vi "Main.vi"() -> ()   [LabVIEW 2020]
doc: "Copyright (c) 2019, Labvolution Limited - www.labvolution.com\n\nThis software is distributed under the BSD 3-Clause License. For the full license please the LICENSE file or visit www.labvolution.com/license"
uses:
  callback-system-exec/CallbackSystemExec.vi
  callback-system-exec/callback-system-exec.lvlib
panel:
  in  "Abort command":bool
  out "Exit":bool
  in  "Execute command":bool
  in  "Working directory":path
  in  "Command":string(combo)
  out "Standard Error":string
  out "Standard Out":string
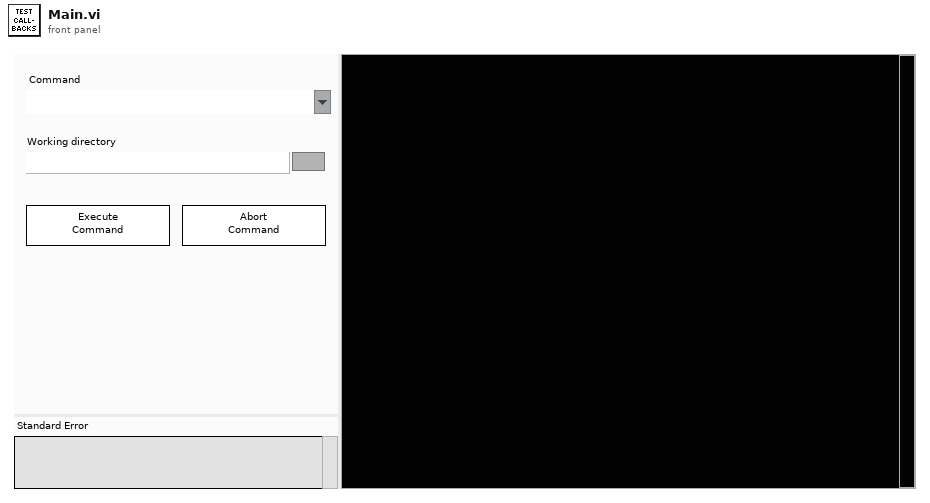
[diagram p1: front panel]
types:
  T1 = cluster{"Standard Out UE":refnum<user-event>, "Standard Error UE":refnum<user-event>, "Exited UE":refnum<user-event>}
  T2 = enum32{"invalid app kind", "Development System", "Run Time System", "Student Edition", "Embedded LabVIEW", "Evaluation", "Custom"}
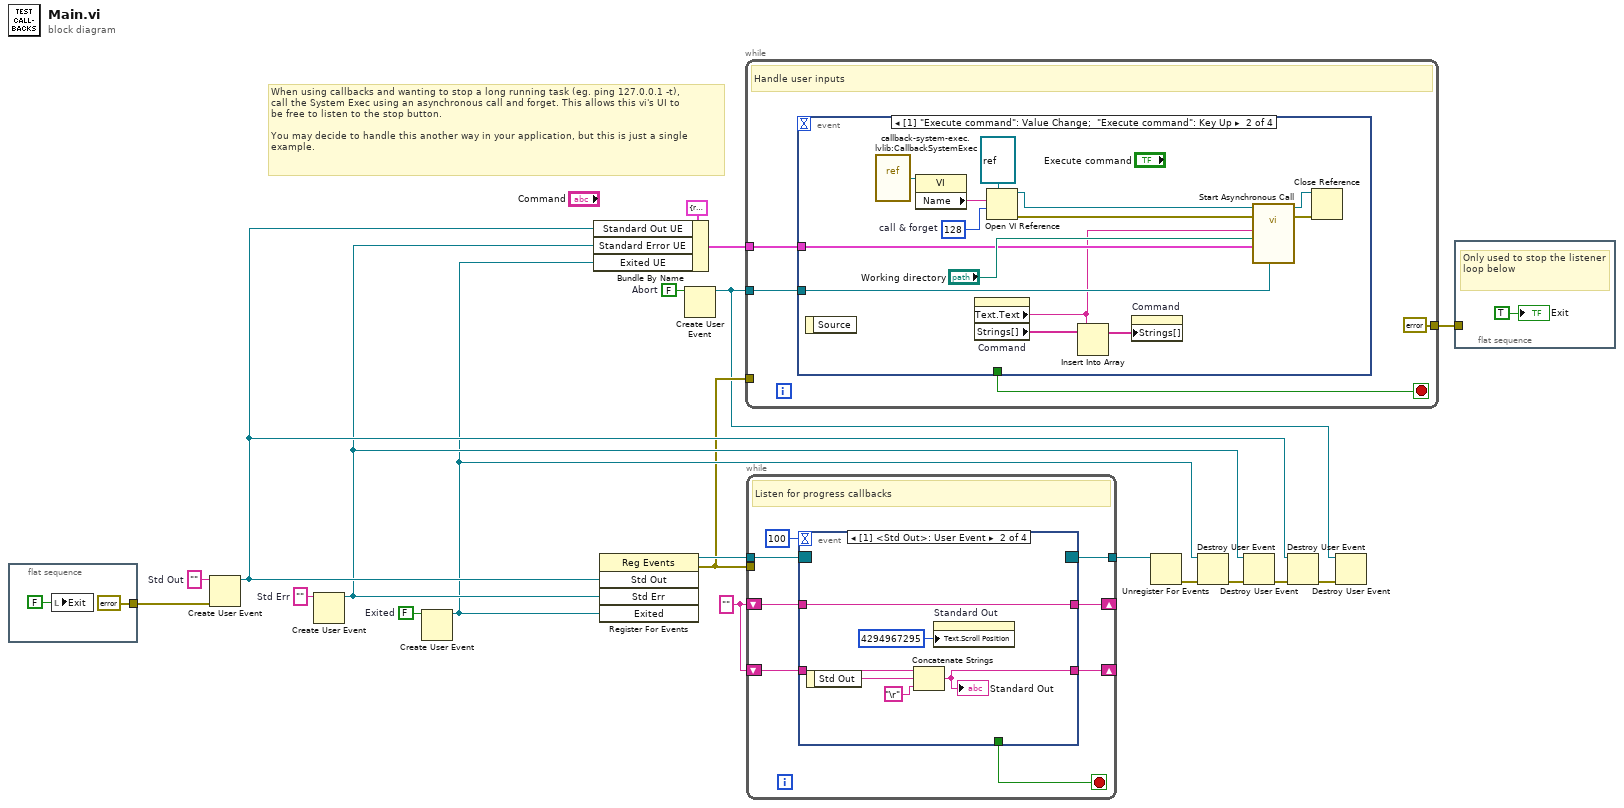
[diagram p0: block diagram]
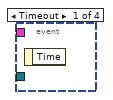
[diagram p2: hidden frame]
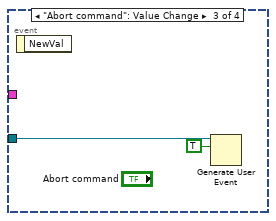
[diagram p3: hidden frame]
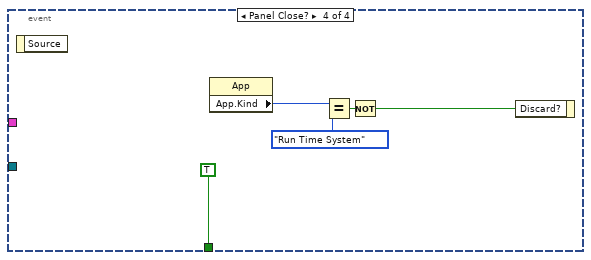
[diagram p4: hidden frame]
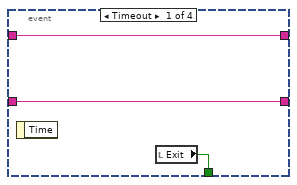
[diagram p5: hidden frame]
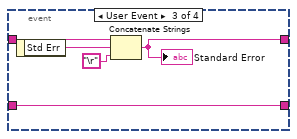
[diagram p6: hidden frame]
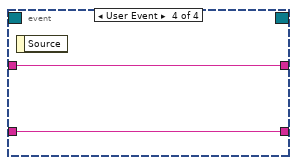
[diagram p7: hidden frame]
diagram:
  w3 = FALSE  # Abort
  w16 = ""
  w20 = FALSE  # Exited
  w19 = ""  # Std Err
  w18 = ""  # Std Out
  # "When using callbacks and wanting to stop a long running task (eg. ping 127.0.0.1 -t),\ncall the System Exec using an asynchronous call and forget. This allows this vi's UI to\nbe free to listen to the stop button.\n\nYou may decide to handle this another way in your application, but this is just a single\nexample."
  n1 = flat-sequence {
    tunnel: [errorcluster {"status"=FALSE, "code"=0, "source"=""} ("error in (no error)")] -> w7
    frame #0 {
      n2 = local write "Exit"(FALSE ("Exit")) -> ()
    }
  }
  n3 = Create User Event(user event datatype=w18, error in=w7) -> (user event=w11:refnum<user-event>)  [unwired: 1 out]
  n4 = Create User Event(user event datatype=w19) -> (user event=w10:refnum<user-event>)  [unwired: 1 in, 1 out]
  n5 = Create User Event(user event datatype=w20) -> (user event=w9:refnum<user-event>)  [unwired: 1 in, 1 out]
  n6 = Bundle By Name(cluster=T1 {"Standard Out UE"=refnum, "Standard Error UE"=refnum, "Exited UE"=refnum} ("Caller Events"), "Standard Out UE"=w11, "Standard Error UE"=w10, "Exited UE"=w9) -> (w4:T1)
  n7 = register-events(w11, w10, w9) -> (reference out=w8:refnum<event-registration>, error out=w6:errorcluster)  [unwired: 2 in]
  n8 = Create User Event(user event datatype=w3) -> (user event=w1:refnum<user-event>)  [unwired: 1 in, 1 out]
  n9 = while {
    tunnel: w4 -> [w25]
    tunnel: w6 -> [_]
    tunnel: [errorcluster {"status"=FALSE, "code"=0, "source"=""} ("error in (no error)")] -> w5
    tunnel: w1 -> [w23]
    stop <- w26 stop-if-true
    # "Handle user inputs"
    n10 = event shown="[1] \"Execute command\": Value Change;  \"Execute command\": Key Up" {
      selector: _ -> [_ _ _ _]
      dyn-events: _ -> [_ _ _ _]
      timeout: _ -> [_ _ _ _]
      tunnel: [_ _ _ TRUE] -> w26
      tunnel: w25 -> [_ w33 _ _]
      tunnel: w23 -> [_ w32 w42 _]
      event Timeout {
        n11 = event-data() -> ()  [unwired: 1 in, 1 out]
      }
      event "Execute command": Value Change; "Execute command": Key Up {
        w36 = 128  # call & forget
        n12 = event-data() -> ()  [unwired: 1 in, 1 out]
        n13 = vi-ref "callback-system-exec.lvlib:CallbackSystemExec.vi"() -> (w38:refnum<vi>)
        n14 = property class="VI"(reference=w38) -> ("Name"=w37:string)  [unwired: 1 in, 2 out]
        n15 = property on="Command" class="CmbBox"() -> ("Text.Text"=w28:string, "Strings[]"=w29:string[])  [unwired: 2 in, 2 out]
        n16 = Open VI Reference(type specifier VI Refnum (for type only)=refnum<vi> refnum, vi path=w37, options=w36) -> (vi reference=w39:refnum<vi>, error out=w40:errorcluster)  [unwired: 3 in]
        n17 = Insert Into Array(array=w29, new element=w28) -> (w27:string[])  [unwired: 1 in]
        n18 = property on="Command" class="CmbBox"("Strings[]"=w27) -> ()  [unwired: 2 in, 2 out]
        n19 = call-by-ref "Start Asynchronous Call"(reference=w39, error in=w40, "Abort UE"=w32, "Caller Events"=w33, "Working directory"="Working directory", "Command"=w28) -> (reference out=w30:refnum<vi>, error out=w31:errorcluster)  [unwired: 5 in, 3 out]
        n20 = Close Reference(reference=w30, error in (no error)=w31) -> ()  [unwired: 1 out]
      }
      event "Abort command": Value Change {
        n21 = event-data() -> ()  [unwired: 1 in, 1 out]
        n22 = Generate User Event(user event=w42, event data cluster=TRUE ("event data")) -> ()  [unwired: 2 in, 2 out]
      }
      event Panel Close? {
        n23 = event-data() -> ()  [unwired: 1 in, 1 out]
        n24 = property class="App"() -> ("App.Kind"=w46:T2)  [unwired: 2 in, 2 out]
        n25 = Equal?(x=w46, y=T2."Run Time System") -> (x = y?=w44:bool)
        n26 = Not(x=w44) -> (.not. x?=w43:bool)
        n27 = event-data("Discard?"=w43) -> ()  [unwired: 1 in, 1 out]
      }
    }
  }
  n28 = while {
    tunnel: [w54] -> w12
    shift-right: [w52] -> _
    shift-left: w16 -> [w53]
    shift-right: [w51] -> _
    shift-left: w16 -> [w50]
    tunnel: w8 -> [w49]
    tunnel: w6 -> [_]
    stop <- w55 stop-if-true
    # "Listen for progress callbacks"
    n29 = event shown="[1] <Std Out>: User Event" {
      selector: w49 -> [_ _ _ _]
      dyn-events: [_ _ _ _] -> w54
      timeout: 100 -> [_ _ _ _]
      tunnel: [w56 _ _ _] -> w55
      tunnel: w53 -> [w57 w63 w69 w71]
      tunnel: [w57 w60 w69 w71] -> w52
      tunnel: [w58 w61 w65 w70] -> w51
      tunnel: w50 -> [w58 w61 w67 w70]
      event Timeout {
        n30 = event-data() -> ()  [unwired: 1 in, 1 out]
        n31 = local read "Exit"() -> (w56:bool)
      }
      event User Event {
        n32 = event-data() -> ("Std Out"=w62:string)  [unwired: 1 in]
        n33 = Concatenate Strings(w63, w62, "\r") -> (w60:string)
        "Standard Out" <- w60
        n34 = property on="Standard Out" class="Str"("Text.Scroll Position"=u32 4294967295) -> ()  [unwired: 2 in, 2 out]
      }
      event User Event {
        n35 = event-data() -> ("Std Err"=w66:string)  [unwired: 1 in]
        n36 = Concatenate Strings(w67, w66, "\r") -> (w65:string)
        "Standard Error" <- w65
      }
      event User Event {
        n37 = event-data() -> ()  [unwired: 1 in, 1 out]
      }
    }
  }
  n38 = Unregister For Events(event registration refnum=w12) -> (error out=w13:errorcluster)  [unwired: 1 in]
  n39 = Destroy User Event(user event=w9, error in=w13) -> (error out=w14:errorcluster)
  n40 = Destroy User Event(user event=w10, error in=w14) -> (error out=w15:errorcluster)
  n41 = Destroy User Event(user event=w11, error in=w15) -> (error out=w2:errorcluster)
  n42 = Destroy User Event(user event=w1, error in=w2) -> ()  [unwired: 1 out]
  n43 = flat-sequence {
    tunnel: w5 -> [_]
    frame #0 {
      # "Only used to stop the listener loop below"
      "Exit" <- TRUE ("Exit")
    }
  }
